vi "队列测试.vi"() -> ()   [LabVIEW 2019, in "test.lvlib"]
uses:
  test.lvlib
panel:
  out "数值":i32
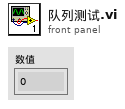
[diagram p1: front panel]
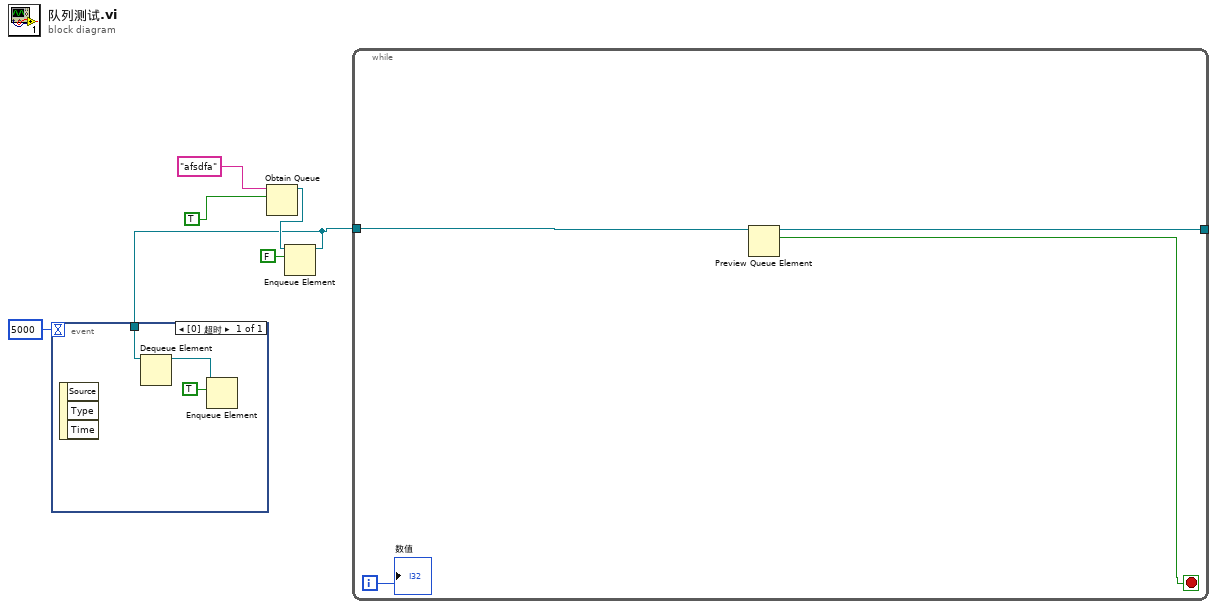
[diagram p0: block diagram]
diagram:
  n1 = Obtain Queue(name (unnamed)="afsdfa" ("名称（未命名）"), element data type=TRUE) -> (queue out=w4:refnum<queue>)  [unwired: 3 in, 2 out]
  n2 = Enqueue Element(queue=w4, element=FALSE ("元素")) -> (queue out=w1:refnum<queue>)  [unwired: 2 in, 2 out]
  n3 = event shown="[0] 超时" {
    selector: _ -> [_]
    dyn-events: _ -> [_]
    timeout: 5000 -> [_]
    tunnel: w1 -> [w9]
    event Timeout {
      n4 = event-data() -> ()  [unwired: 1 in, 3 out]
      n5 = Dequeue Element(queue=w9) -> (queue out=w8:refnum<queue>)  [unwired: 2 in, 3 out]
      n6 = Enqueue Element(queue=w8, element=TRUE ("元素")) -> ()  [unwired: 2 in, 3 out]
    }
  }
  n7 = while {
    tunnel: w1 -> [w13]
    tunnel: [w11] -> _
    i -> [w10]
    stop <- w12 stop-if-true
    n8 = Preview Queue Element(queue=w13) -> (queue out=w11:refnum<queue>, element=w12:bool)  [unwired: 2 in, 2 out]
    "数值" <- w10
  }
